vi "CAN 6 SPARK MAX Motor Set Value.vi"(6 "Control Mode":T1, 7 "Velocity Offset":dbl, 9 "Right Power":dbl, 10 "Left Power":dbl, 11 "Drivetrain":T2) -> ()   [LabVIEW 2019]
uses:
  SPARKMAX6Motor.ctl
  <vilib>/Rock Robotics/WPI/MotorControl/WPI_MotorControlDeviceRef.ctl
  <vilib>/Rock Robotics/WPI/MotorControl/WPI_MotorControlType.ctl
  <vilib>/Rock Robotics/SystemInterfaces/DIO/FPGA_DIOPWMChannel.ctl
  <vilib>/Rock Robotics/WPI/PWM/WPI_PWMDeadband.ctl
  <vilib>/Rock Robotics/SystemInterfaces/DIO/FPGA_DIOChannel.ctl
  <vilib>/Rock Robotics/WPI/ThirdParty/REV Robotics/SPARK MAX/Typedef/Spark MAX Control Type.ctl
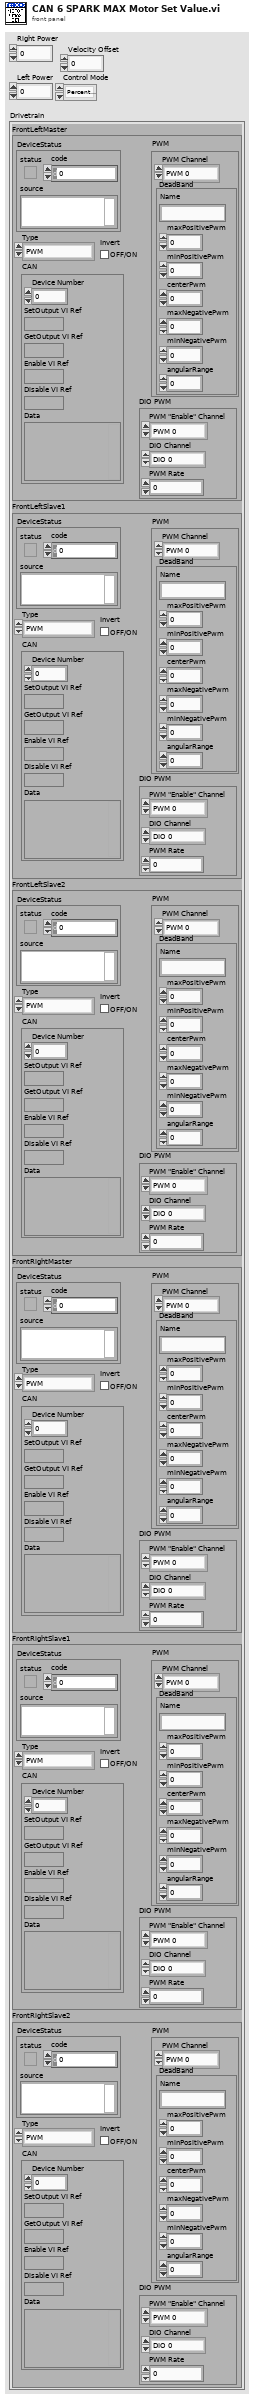
[diagram p1: front panel]
types:
  T1 = typedef "Spark MAX Control Type.ctl" = enum16{"Percent VBus", "Voltage", "Velocity", "Position", "Smart Motion", "Current", "Smart Velocity"}
  T2 = typedef "SPARKMAX6Motor.ctl" = cluster{"FrontLeftMaster":T3, "FrontLeftSlave1":T3, "FrontLeftSlave2":T3, "FrontRightMaster":T3, "FrontRightSlave1":T3, "FrontRightSlave2":T3}
  T3 = typedef "WPI_MotorControlDeviceRef.ctl" = cluster{"DeviceStatus":errorcluster, "Type":T4, "PWM":cluster{"PWM Channel":T5, "DeadBand":T6}, "CAN":cluster{"Device Number":u8, "SetOutput VI Ref":variant, "GetOutput VI Ref":variant, "Enable VI Ref":variant, "Disable VI Ref":variant, "Data":variant}, "Invert":bool, "DIO PWM":cluster{"PWM \"Enable\" Channel":T5, "DIOChannel":T7, "PWM Rate":dbl}}
  T4 = typedef "WPI_MotorControlType.ctl" = enum16{"PWM", "CAN", "DIO PWM"}
  T5 = typedef "FPGA_DIOPWMChannel.ctl" = enum8{"PWM 0", "PWM 1", "PWM 2", "PWM 3", "PWM 4", "PWM 5", "PWM 6", "PWM 7", "PWM 8", "PWM 9", "PWM MXP 0", "PWM MXP 1", "PWM MXP 2", "PWM MXP 3", "PWM MXP 4", "PWM MXP 5", "PWM MXP 6", "PWM MXP 7", "PWM MXP 8", "PWM MXP 9", "Invalid"}
  T6 = typedef "WPI_PWMDeadband.ctl" = cluster{"Name":string, "maxPositivePwm":i32, "minPositivePwm":i32, "centerPwm":i32, "maxNegativePwm":i32, "minNegativePwm":i32, "angularRange":u16}
  T7 = typedef "FPGA_DIOChannel.ctl" = enum8{"DIO 0", "DIO 1", "DIO 2", "DIO 3", "DIO 4", "DIO 5", "DIO 6", "DIO 7", "DIO 8", "DIO 9", "DIO MXP 0", "DIO MXP 1", "DIO MXP 2", "DIO MXP 3", "DIO MXP 4", "DIO MXP 5", "DIO MXP 6", "DIO MXP 7", "DIO MXP 8", "DIO MXP 9", "DIO MXP 10", "DIO MXP 11", "DIO MXP 12", "DIO MXP 13", "DIO MXP 14", "DIO MXP 15", "SPI Port CS1", "SPI Port CS2", "SPI Port CS3", "SPI Port MISO", "SPI Port MOSI", "Invalid"}
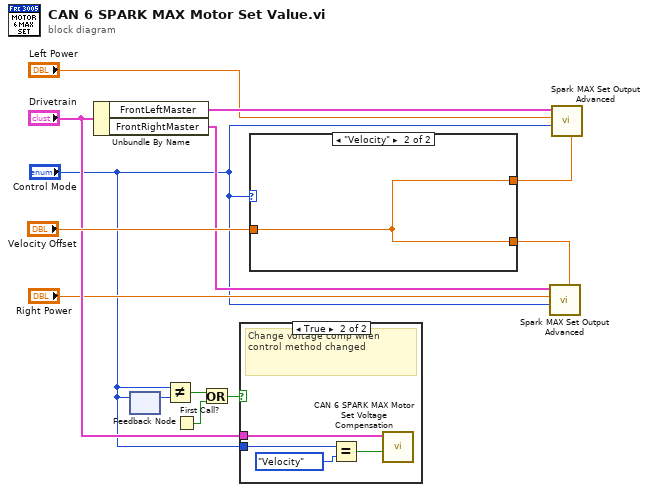
[diagram p0: block diagram]
diagram:
  n1 = Unbundle By Name("Drivetrain") -> ("FrontLeftMaster"=w4:T3, "FrontRightMaster"=w7:T3)
  n2 = feedback-in #1("Control Mode") -> ()
  n3 = feedback #1() -> (w8:T1)  [unwired: 1 in]
  n4 = Not Equal?(x="Control Mode", y=w8) -> (x != y?=w11:bool)
  n5 = First Call?() -> (First Call?: T/F=w9:bool)
  n6 = Or(x=w11, y=w9) -> (x .or. y?=w10:bool)
  n7 = case shown="True" w10 {
    tunnel: "Drivetrain" -> [_ w17]
    tunnel: "Control Mode" -> [_ w16]
    frame False {
    }
    frame True {
      # "Change voltage comp when control method changed"
      n8 = Equal?(x=w16, y=Spark_MAX_Control_Type."Velocity") -> (x = y?=w15:bool)
      n9 = call "CAN 6 SPARK MAX Motor Set Voltage Compensation.vi"("Enable? (F)"=w15, "TalonSRX6MotorRef"=w17) -> ()  [unwired: 9 in, 1 out]
    }
  }
  n10 = case shown="\"Velocity\"" "Control Mode" {
    tunnel: "Velocity Offset" -> [_ w18]
    tunnel: [_ w18] -> w1
    tunnel: [_ w18] -> w5
    frame "Percent VBus", Default {
    }
    frame "Velocity" {
    }
  }
  n11 = call <vilib>:"Spark MAX Set Output Advanced.vi"("Arbitrary Feed Forward (0)"=w5, "Control Mode"="Control Mode", "Setpoint"="Right Power", "MotorControlDevRef"=w7) -> ()  [unwired: 6 in, 2 out]
  n12 = call <vilib>:"Spark MAX Set Output Advanced.vi"("Arbitrary Feed Forward (0)"=w1, "Control Mode"="Control Mode", "Setpoint"="Left Power", "MotorControlDevRef"=w4) -> ()  [unwired: 6 in, 2 out]
